vi "PWMInit.vi"(8 "ErrorIn(no error)":errorcluster, 10 "PMWFreq(200Hz)":u32=200, 11 "FPGA VI引用输入":refnum<k20>) -> (0 "ErrorOut":errorcluster, 3 "FPGA VI引用输出":refnum<k20>)   [LabVIEW 2015]
uses:
  <vilib>/Utility/error.llb/Error Cluster From Error Code.vi
  <vilib>/rvi/errors/niLvFpgaAdjustHostInterfaceError.vi
  <vilib>/rvi/interface/nirviReadWriteControl/nirviReadWriteControl.xnode
  NiFpgaLv.dll
  <vilib>/rvi/interface/Simulation/niFpgaSimulationCallBeginRW.vi
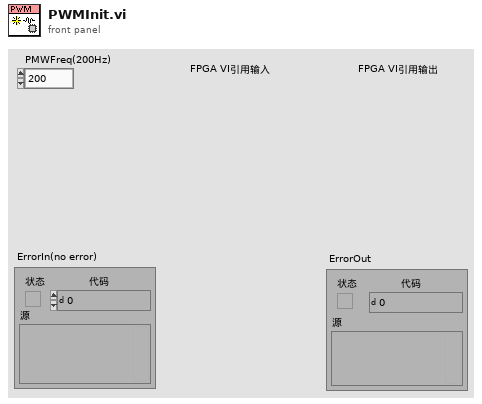
[diagram p1: front panel]
types:
  T1 = cluster{"PWM0":u16, "PWM1":u16, "PWM2":u16, "PWM3":u16}
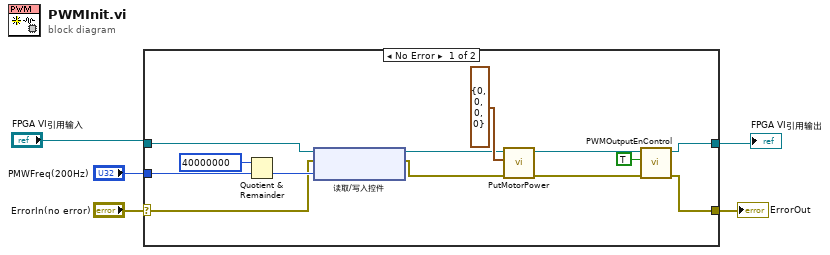
[diagram p0: block diagram]
diagram:
  n1 = case shown="No Error" "ErrorIn(no error)" {
    selector: "ErrorIn(no error)" -> [w14 w19]
    tunnel: "FPGA VI引用输入" -> [w18 w20]
    tunnel: "PMWFreq(200Hz)" -> [w16 _]
    tunnel: [w13 w20] -> w1
    tunnel: [w12 w19] -> w3
    frame No Error {
      n2 = Quotient & Remainder(x=u32 40000000, y=w16) -> (floor(x/y)=w15:u32)  [unwired: 1 out]
      n3 = xnode "读取/写入控件"("FPGA VI Reference In"=w18, "error in"=w14, "CounterMAX"=w15) -> ("FPGA VI Reference Out"=w6:refnum<k20>, "error out"=w8:errorcluster)
      n4 = call "PutMotorPower.vi"("ErrorIn(no error)"=w8, "MotorPower"=T1 {"PWM0"=0, "PWM1"=0, "PWM2"=0, "PWM3"=0}, "FPGA VI引用输入"=w6) -> ("ErrorOut"=w9:errorcluster, "FPGA VI引用输出"=w10:refnum<k20>)  [unwired: 7 in]
      n5 = call "PWMOutputEnControl.vi"("ErrorIn(no error)"=w9, "OutEN?(F)"=TRUE, "FPGA VI引用输入"=w10) -> ("ErrorOut"=w12:errorcluster, "FPGA VI引用输出"=w13:refnum<k20>)  [unwired: 7 in]
    }
    frame Error {
    }
  }
  "ErrorOut" <- w3
  "FPGA VI引用输出" <- w1
